vi "Execute Spurious Emission Page.vi"(0 "VISA resource name":refnum<visa-resource-name>, 5 "Spurious Emission Page (0:Next Page)":i32(ring) items=["Next Page", "Previous Page"], 11 "error in (no error)":errorcluster) -> (4 "VISA resource name out":refnum<visa-resource-name>, 15 "error out":errorcluster)   [LabVIEW 2020, in "Anritsu Signal Analyzer Series.lvlib"]
doc: "Sets the Spurious Emission Page Action\n\nSet Spurious Emission Next Page.\nSet Spurious Emission Previous Page."
uses:
  Anritsu Signal Analyzer Series.lvlib
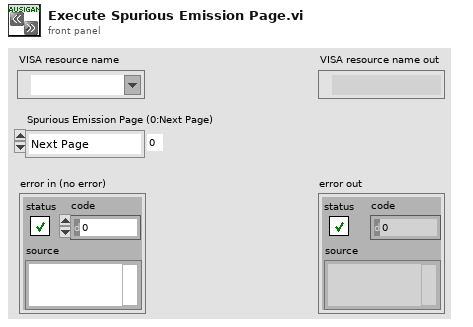
[diagram p1: front panel]
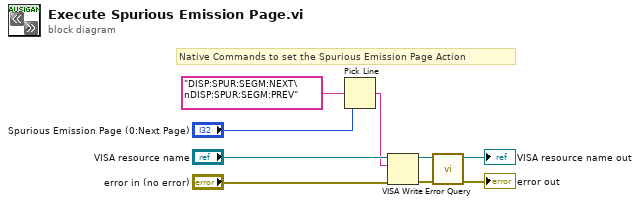
[diagram p0: block diagram]
diagram:
  # "Native Commands to set the Spurious Emission Page Action"
  n1 = Pick Line(multi-line string="DISP:SPUR:SEGM:NEXT\nDISP:SPUR:SEGM:PREV" ("_Command"), line index="Spurious Emission Page (0:Next Page)") -> (output string=w1:string)  [unwired: 1 in]
  n2 = VISA Write(VISA resource name="VISA resource name", write buffer=w1, error in (no error)="error in (no error)") -> (VISA resource name out=w5:refnum<visa-resource-name>, error out=w4:errorcluster)  [unwired: 1 out]
  n3 = call "Error Query.vi"("error in (no error)"=w4, "VISA resource name"=w5) -> ("error out"=→"error out":errorcluster, "VISA resource name out"=→"VISA resource name out":refnum<visa-resource-name>)  [unwired: 6 in, 2 out]
